vi "FindClosestPointOnMove.vi"() -> ()   [LabVIEW 2015]
uses:
  Navigation2017-util.lvlib
  Vector.ctl
  Navigation2017.lvlib
panel:
  out "Closest Vector":T1
  in  "Move Positions":T1[](array[typedef])
  in  "Current Robot Position":T1
  out "Signed Angle Error":dbl
  out "Coordinate Error":dbl
  out "Closest Index":dbl
  in  "Start Index":i32
  # "OUTPUTS"
  # "INPUTS"
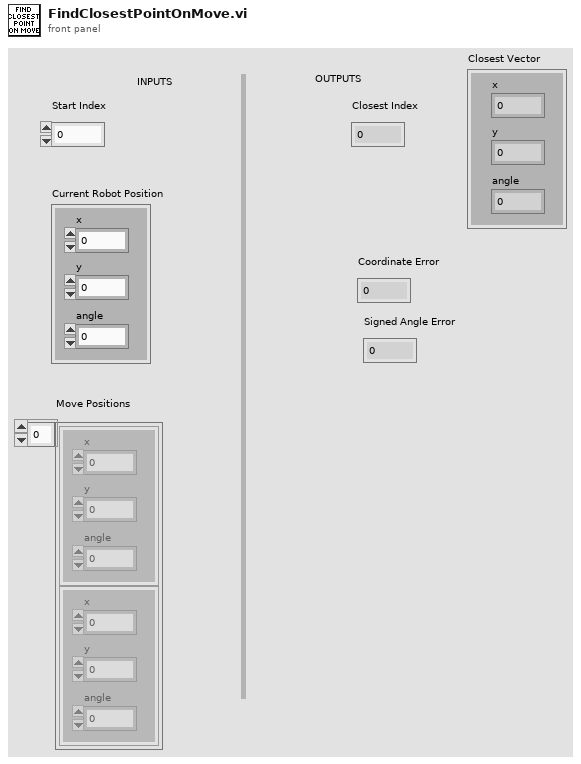
[diagram p1: front panel]
types:
  T1 = typedef "Navigation2017.lvlib/Vector.ctl" = cluster{"x":dbl, "y":dbl, "angle":dbl}
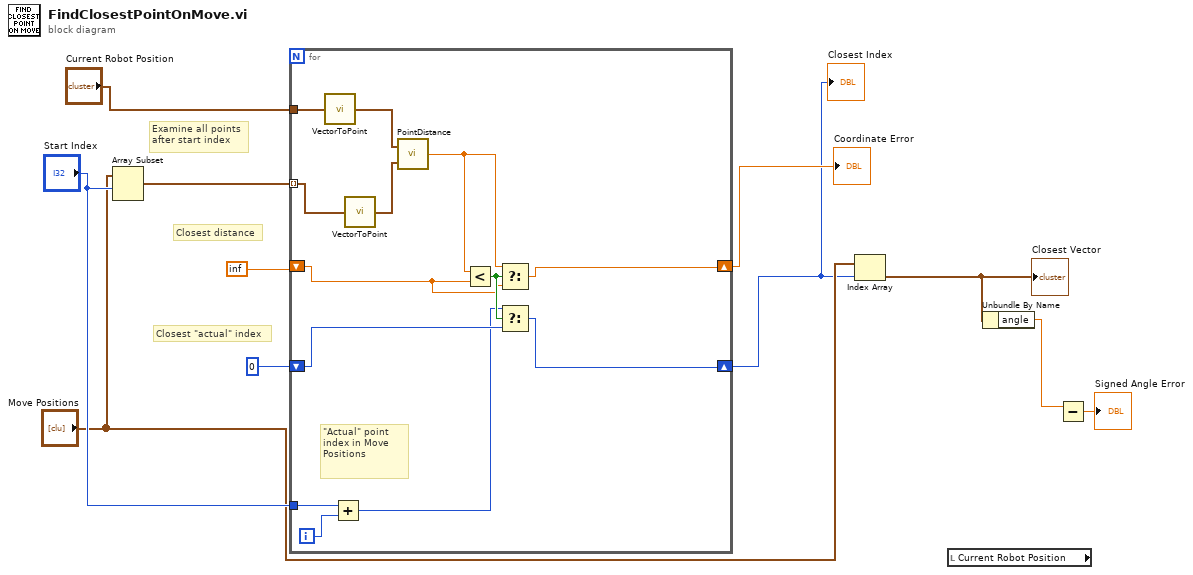
[diagram p0: block diagram]
diagram:
  # "Closest \"actual\" index"
  # "Closest distance"
  # "Examine all points\nafter start index"
  n1 = Array Subset(array="Move Positions", index="Start Index") -> (w11:T1[])  [unwired: 1 in]
  n2 = for {
    tunnel: w11 -> [w22] mode=indexing
    tunnel: "Start Index" -> [w23]
    tunnel: "Current Robot Position" -> [w19]
    shift-right: [w15] -> w6
    shift-left: inf -> [w16]
    shift-right: [w14] -> w4
    shift-left: 0 -> [w17]
    i -> [w24]
    # "\"Actual\" point index in Move Positions"
    n3 = call "VectorToPoint.vi"("Vector"=w19) -> ("Point"=w20:cluster{"x":dbl, "y":dbl})
    n4 = Add(x=w23, y=w24) -> (x+y=w13:i32)
    n5 = call "VectorToPoint.vi"("Vector"=w22) -> ("Point"=w21:cluster{"x":dbl, "y":dbl})
    n6 = call "PointDistance.vi"("Point 2"=w21, "Point 1"=w20) -> ("Distance"=w12:dbl)
    n7 = Less?(x=w12, y=w16) -> (x < y?=w18:bool)
    n8 = Select(t=w12, s=w18, f=w16) -> (s? t:f=w15:dbl)
    n9 = Select(t=w13, s=w18, f=w17) -> (s? t:f=w14:i32)
  }
  "Closest Index" <- w4
  "Coordinate Error" <- w6
  n10 = Index Array(array="Move Positions", index=w4) -> (element=w2:T1)
  "Closest Vector" <- w2
  n11 = local read "Current Robot Position"() -> ()  [unwired: 1 out]
  n12 = Unbundle By Name(w2) -> ("angle"=w1:dbl)
  n13 = Subtract(x=w1) -> (x-y=→"Signed Angle Error":dbl)  [unwired: 1 in]
